vi "Set Server gRPC UEs.vi"(10 "Server gRPC UEs":T1, 11 "OOP Server in":refnum<class "helloWServer.lvclass">) -> (3 "OOP Server out":refnum<class "helloWServer.lvclass">)   [LabVIEW 2020, in "helloWServer.lvlib" / "helloWServer.lvclass"]
uses:
  helloWServer.lvclass
  typeDefs/Server gRPC UEs.ctl
  helloWServer.lvclass/helloWServer.ctl
  gRPC lvSupport/Server API/typeDefs/grpcId.ctl
  gRPC lvSupport/gprc-lvsupport.lvlib
  gRPC lvSupport/Server API/typeDefs/gRPCId Cluster.ctl
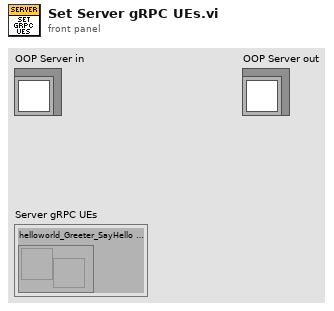
[diagram p1: front panel]
types:
  T1 = typedef "helloWServer.lvlib/helloWServer.lvclass/Server gRPC UEs.ctl" = cluster{"helloworld_Greeter_SayHello gRPC UE":refnum<user-event>}
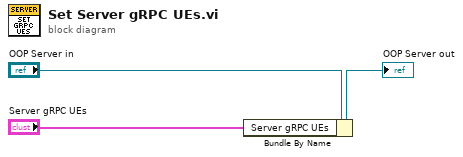
[diagram p0: block diagram]
diagram:
  n1 = Bundle By Name(cluster="OOP Server in", "Server gRPC UEs"="Server gRPC UEs") -> (→"OOP Server out":refnum<class "helloWServer.lvclass">)
